vi "Check if serial numebr is in Database.vi"(0 "connection reference":T1, 5 "table":string, 7 "Serial Number":string, 11 "error in (no error)":errorcluster) -> (4 "connection reference out":T1, 6 "NumberOfTests":string, 8 "Can test":bool, 10 "Device Passed Previous testing":bool, 15 "error out":errorcluster)   [LabVIEW 2023, in "SQL Database.lvlib"]
uses:
  SQL Database.lvlib
  <vilib>/addons/database/Connection.llb/Conn ObjectReference.ctl
  <vilib>/addons/database/_DB Variant To Data/Database Variant To Data.xnode
  <vilib>/addons/database/NI_Database_API.lvlib
panel:
  out "data":variant[][](array[variant])
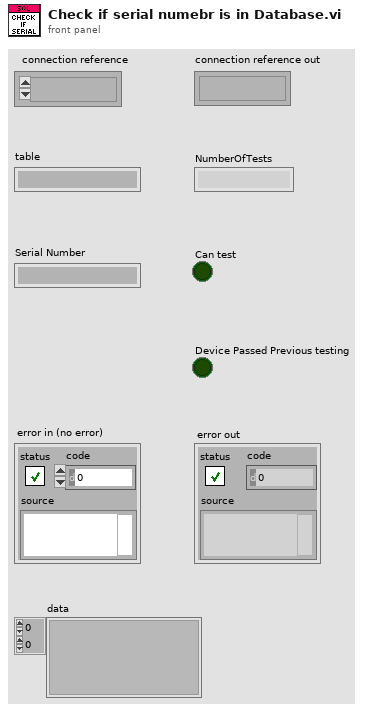
[diagram p1: front panel]
types:
  T1 = typedef "NI_Database_API.lvlib/Conn ObjectReference.ctl" = refnum<k1>
  T2 = cluster{"SerialNumber":string, "NumberOfTests":string, "TestingStatus":string}
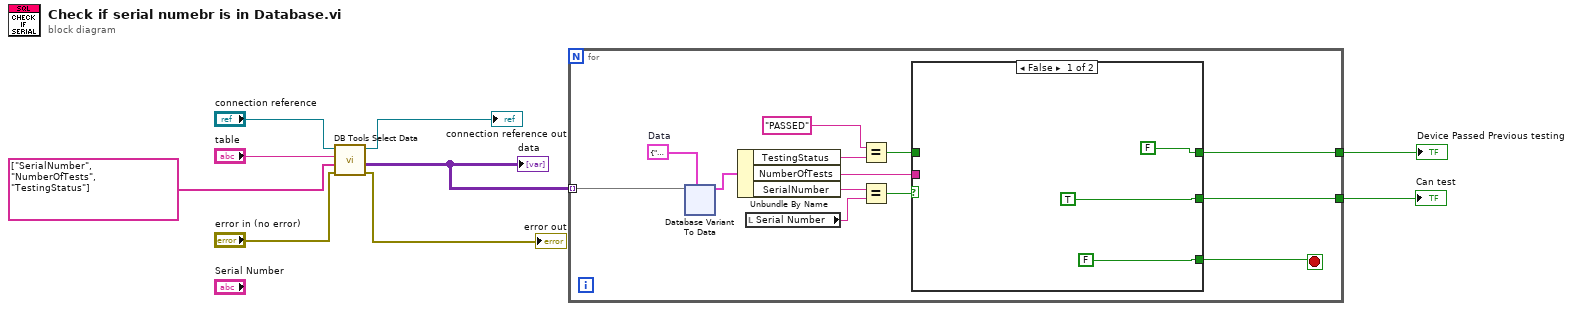
[diagram p0: block diagram]
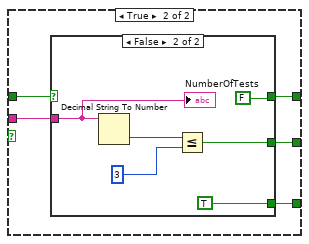
[diagram p2: hidden frame]
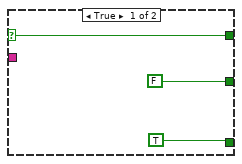
[diagram p3: hidden frame]
diagram:
  n1 = call <vilib>:"DB Tools Select Data.vi"("error in (no error)"="error in (no error)", "columns"=string[] ["SerialNumber", "NumberOfTests", "TestingStatus"], "table"="table", "connection reference"="connection reference") -> ("error out"=→"error out":errorcluster, "data"=w3:variant[][], "connection reference out"=→"connection reference out":T1)  [unwired: 2 in]
  "data" <- w3
  n2 = for {
    tunnel: w3 -> [w22] mode=indexing
    tunnel: [w17] -> w2
    tunnel: [w10] -> w1
    stop <- w16 stop-if-true
    w15 = T2 {"SerialNumber"="", "NumberOfTests"="", "TestingStatus"=""}  # Data
    n3 = xnode "Database Variant To Data"("database variant"=w22, "type"=w15) -> ("data"=w14:T2)  [unwired: 1 in, 1 out]
    n4 = Unbundle By Name(w14) -> ("TestingStatus"=w12:string, "NumberOfTests"=w18:string, "SerialNumber"=w21:string)
    n5 = local read "Serial Number"() -> (w20:string)
    n6 = Equal?(x="PASSED" ("TestingStatus"), y=w12) -> (x = y?=w11:bool)
    n7 = Equal?(x=w21, y=w20) -> (x = y?=w19:bool)
    n8 = case shown="False" w19 {
      tunnel: w18 -> [_ w28]
      tunnel: [TRUE w29] -> w17
      tunnel: [FALSE w30] -> w16
      tunnel: w11 -> [_ w27]
      tunnel: [FALSE w26] -> w10
      frame False {
      }
      frame True {
        n9 = case shown="False" w27 {
          selector: w27 -> [w33 _]
          tunnel: [TRUE TRUE] -> w30
          tunnel: [FALSE w36] -> w29
          tunnel: w28 -> [_ w35]
          tunnel: [w33 FALSE] -> w26
          frame True {
          }
          frame False {
            n10 = Decimal String To Number(string=w35) -> (number=w38:i32)  [unwired: 2 in, 1 out]
            n11 = Less Or Equal?(x=w38, y=3) -> (x <= y?=w36:bool)
            "NumberOfTests" <- w35
          }
        }
      }
    }
  }
  "Can test" <- w2
  "Device Passed Previous testing" <- w1
